vi "Help Page Mech.vi"() -> ()   [LabVIEW 2013]
panel:
  in  "OK Button":bool
  # "To be added: Directions to use the mechanic interruption analysis program"
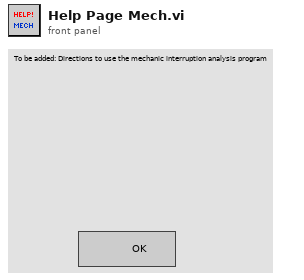
[diagram p1: front panel]
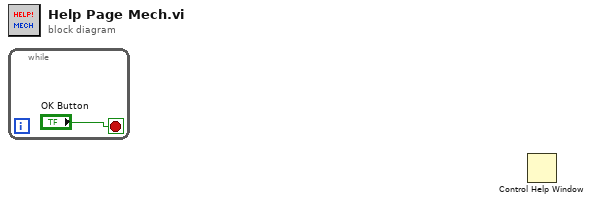
[diagram p0: block diagram]
diagram:
  n1 = while {
    stop <- "OK Button" stop-if-true
  }
  n2 = Control Help Window() -> ()  [unwired: 2 in]
